vi "FileBLFOpen.vi"(6 "提示语":refnum<vi>, 7 "Language":u32, 8 "进度条":refnum<vi>, 9 "进度数值":refnum<vi>, 10 "报文行数统计":refnum<vi>, 11 "file path (dialog if empty)":path caption="文件路径 （空时为对话框）") -> (0 "路径输出":path, 1 "重构的Data数组":u32[][](array[numeric]), 2 "统计数量":string[](array[string]), 3 "报文ID":string[](array[string]), 4 "基时间簇":T1 {"基时间秒" format="%#.6f"}, 5 "CAN报文统计":string[][](array[string]))   [LabVIEW 2015]
uses:
  BLF/Read Write BLF.lvclass/Read Write BLF.ctl
  GetBinlogdllpath.vi
  BasicAppPath.vi
  <vilib>/Utility/libraryn.llb/Check if File or Folder Exists.vi
  <vilib>/Utility/error.llb/Error Cluster From Error Code.vi
  BLF/Read Write BLF.lvclass
panel:
  out "Object Count":u32
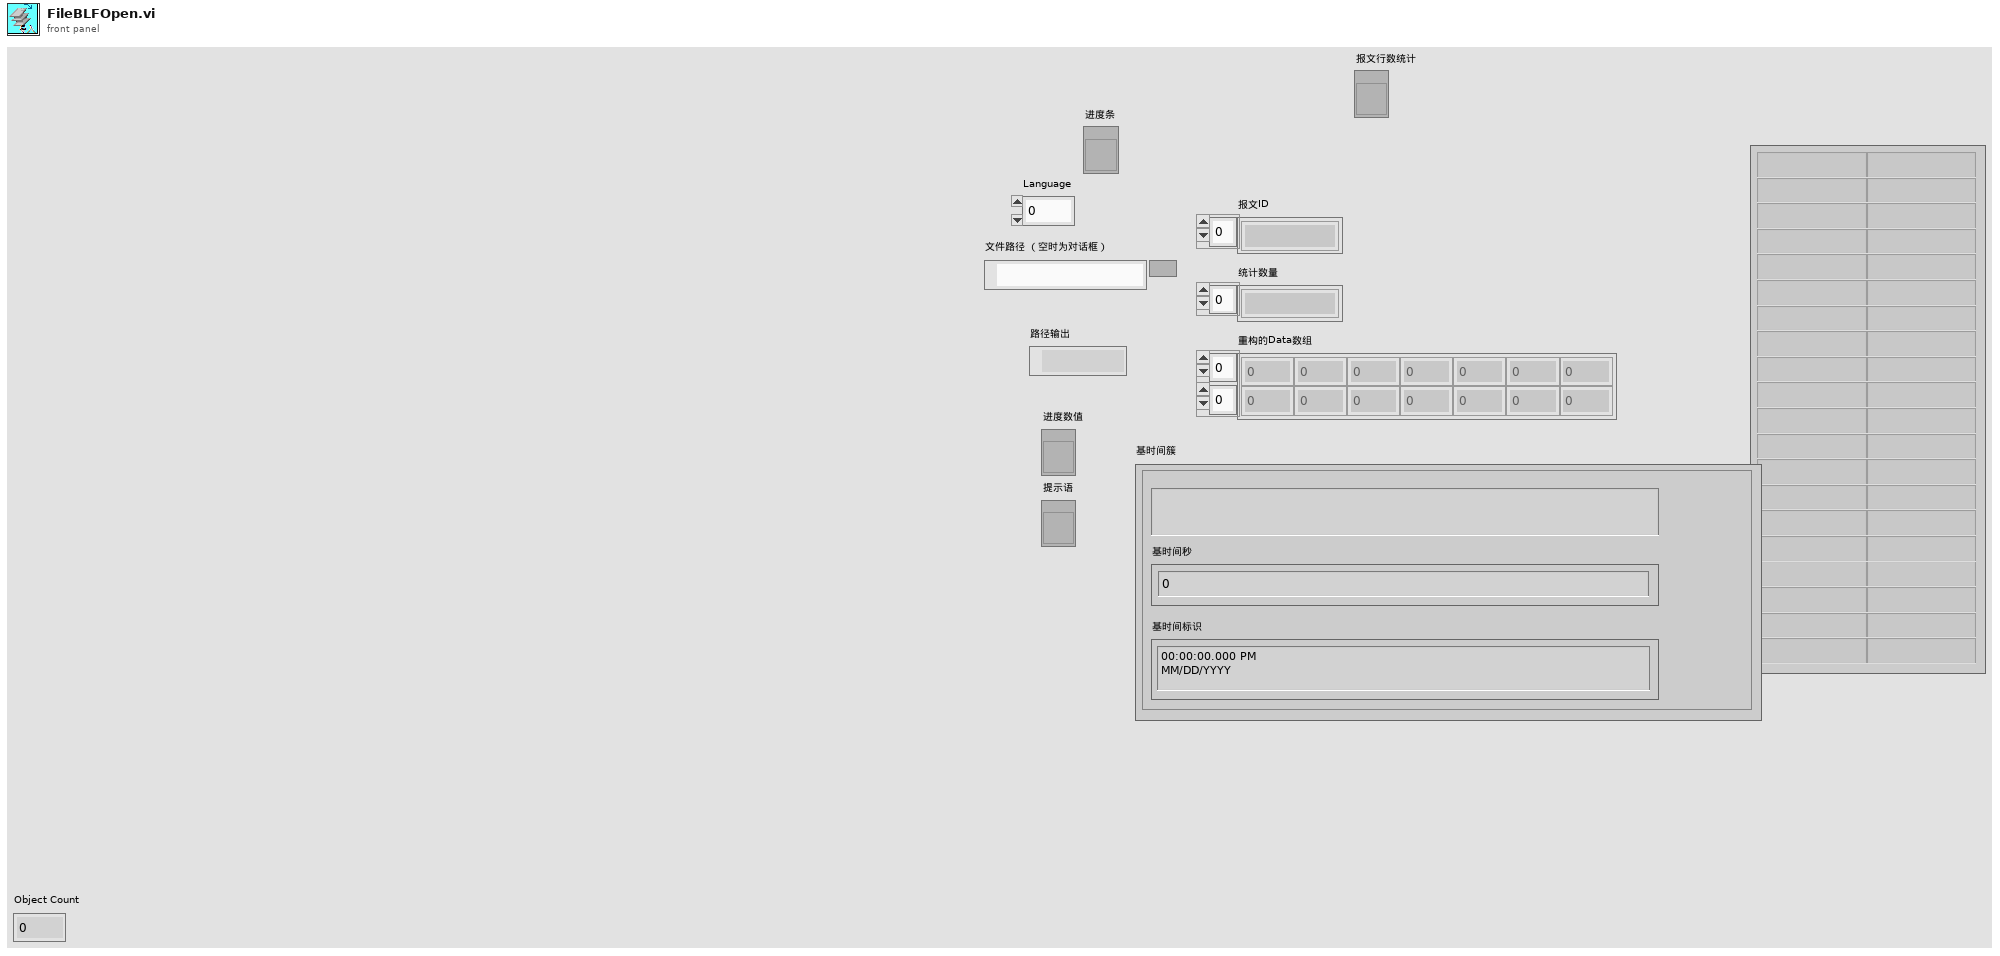
[diagram p1: front panel]
types:
  T1 = cluster{"基时间字符串":string, "基时间秒":dbl, "基时间标识":timestamp}
  T2 = typedef "Read Write BLF.lvclass/Cluster - CAN Frame.ctl" = cluster{"timestamp":timestamp, "payload":u8[], "identifier":u32, "extended?":bool, "echo?":bool, "type":T3}
  T3 = typedef "Read Write BLF.lvclass/Enum - CAN Data Type.ctl" = u8
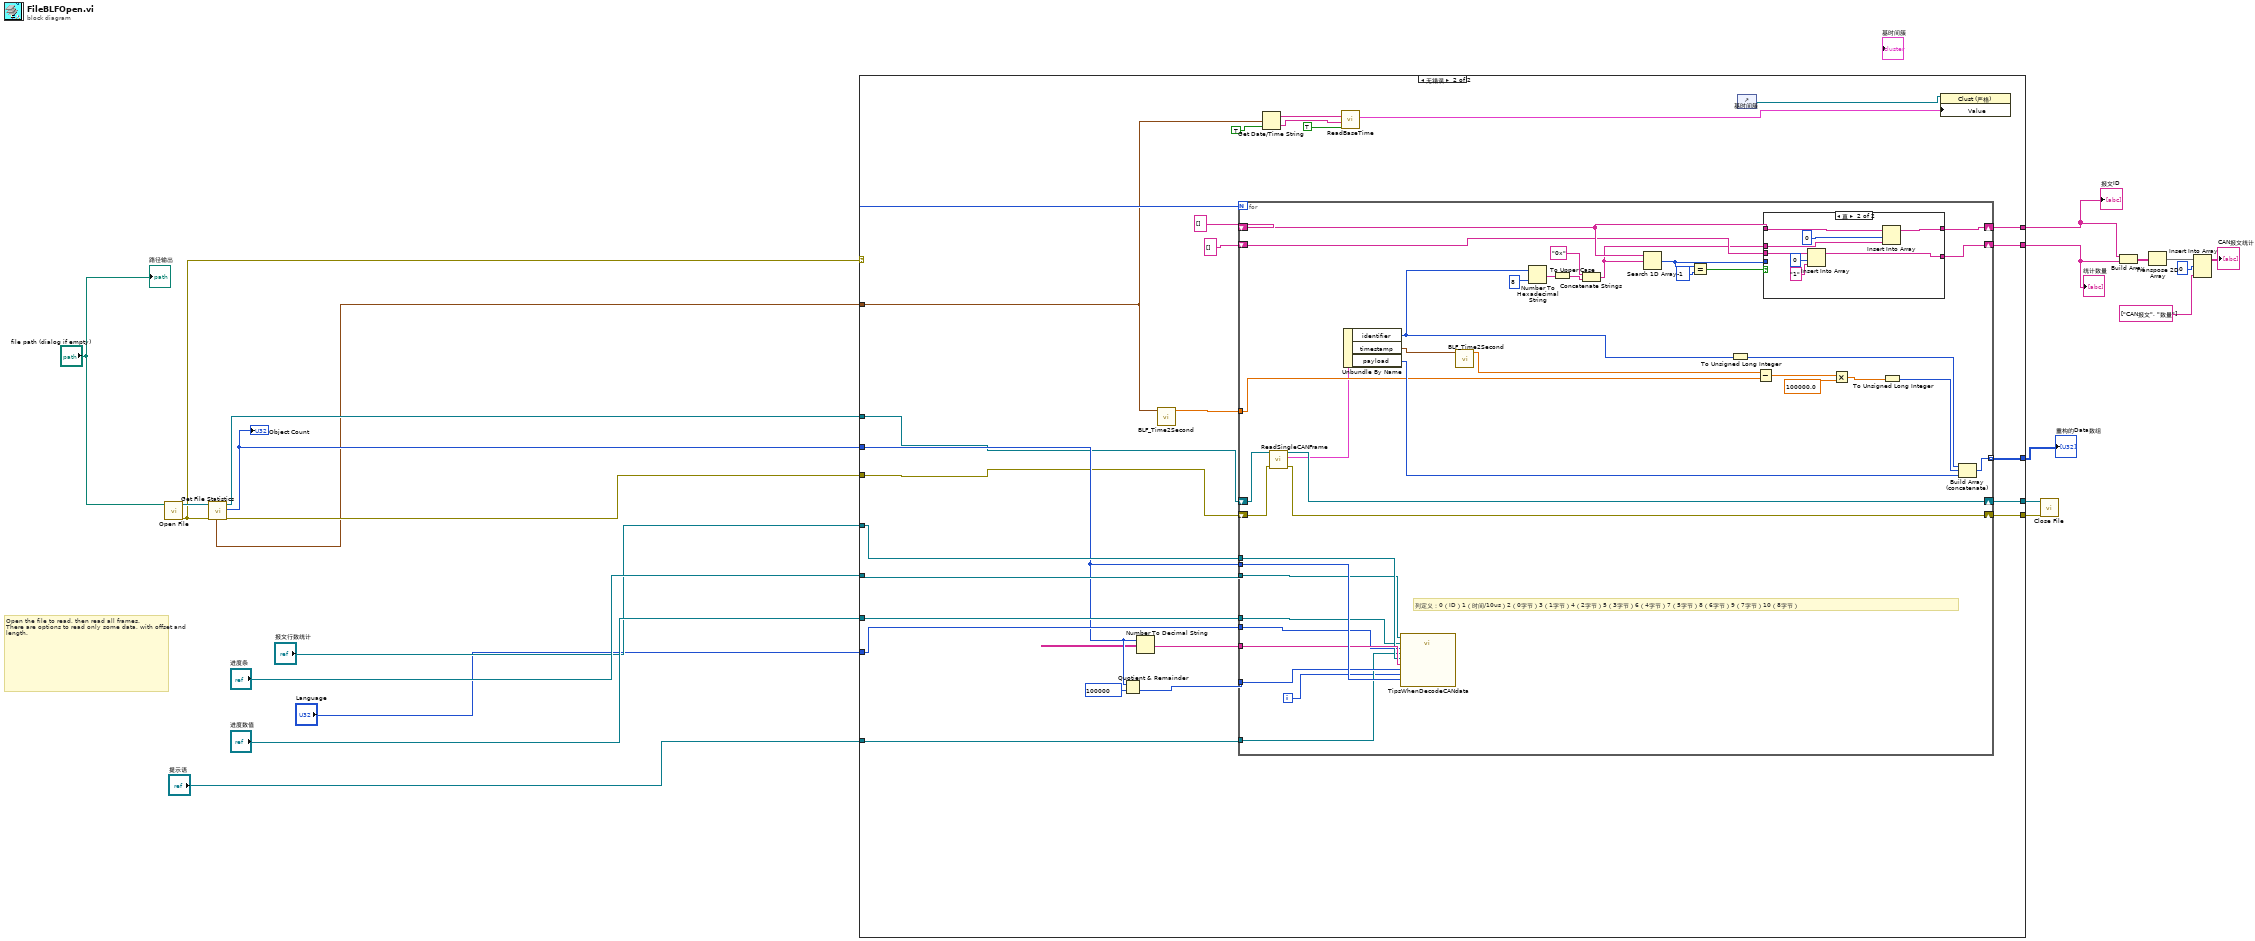
[diagram p0: block diagram]
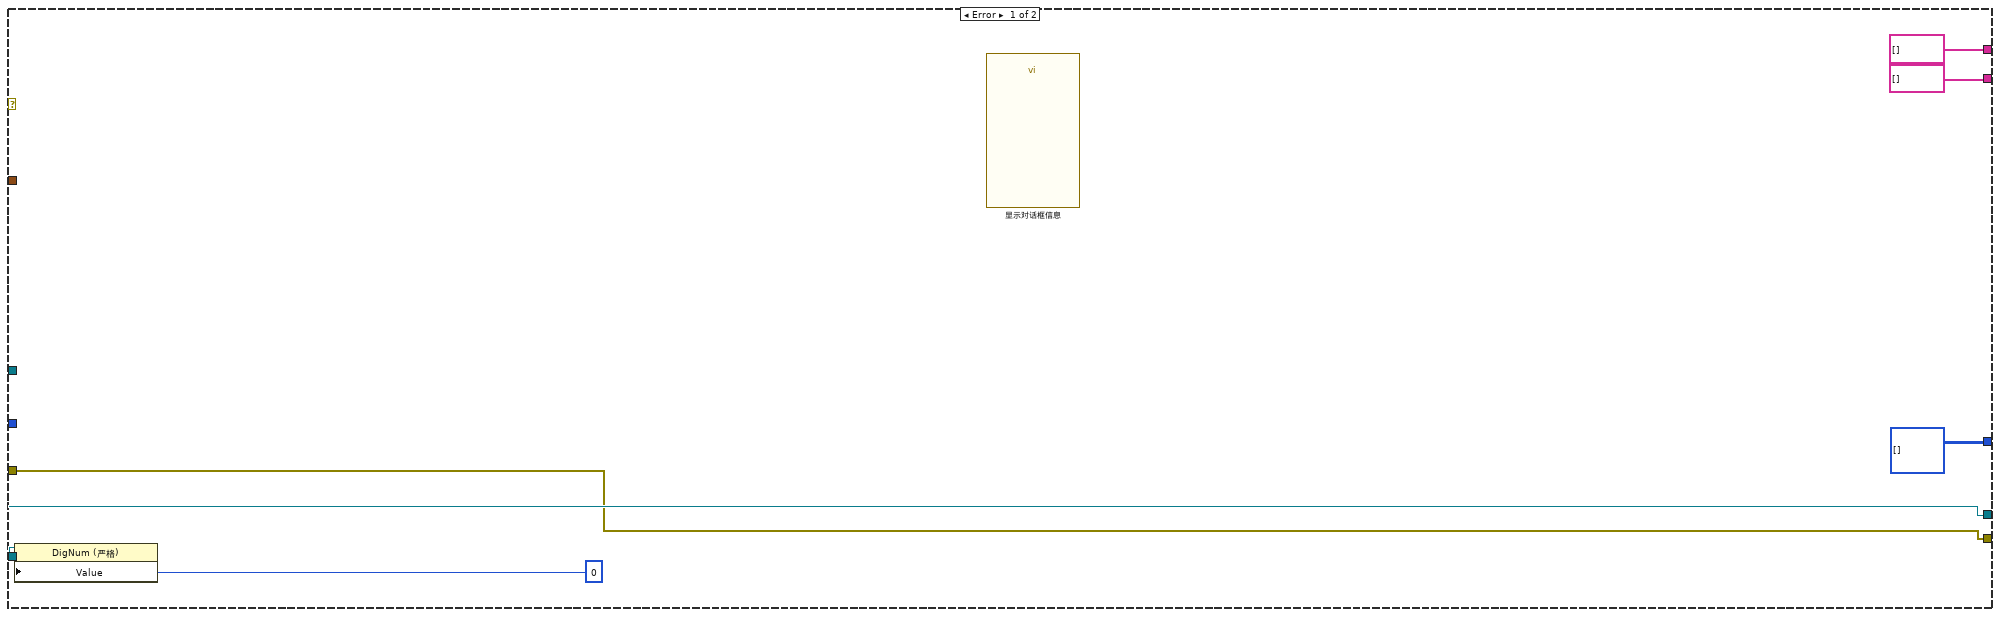
[diagram p2: hidden frame]
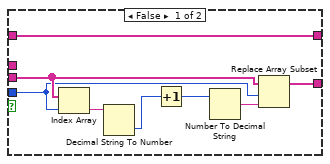
[diagram p3: hidden frame]
diagram:
  # "Open the file to read, then read all frames.\nThere are options to read only some data, with offset and length."
  n1 = call "Open File.vi"("Log Path"="file path (dialog if empty)") -> ("error out"=w8:errorcluster, "BLF File"=w10:refnum<class "Read Write BLF.lvclass">)  [unwired: 9 in]
  n2 = call "Get File Statistics.vi"("error in (no error)"=w8, "Read Write BLF in"=w10) -> ("error out"=w4:errorcluster, "Object Count"=w6:u32, "Read Write BLF out"=w5:refnum<class "Read Write BLF.lvclass">, "Start Time"=w3:timestamp)  [unwired: 3 in, 3 out]
  "Object Count" <- w6
  n3 = case shown="无错误" w8 {
    tunnel: [u32[][] [] w55] -> w22
    tunnel: [string[] [] w52] -> w17
    tunnel: [string[] [] w51] -> w16
    tunnel: "进度条" -> [_ w50]
    tunnel: "进度数值" -> [_ w49]
    tunnel: "提示语" -> [_ w37]
    tunnel: "报文行数统计" -> [w26 w45]
    tunnel: "Language" -> [_ w44]
    tunnel: w6 -> [_ w43]
    tunnel: w5 -> [w24 w32]
    tunnel: w4 -> [w23 w30]
    tunnel: w3 -> [_ w34]
    tunnel: [w24 w33] -> w2
    tunnel: [w23 w31] -> w1
    frame Error {
      n4 = property class="DigNum (严格)"(reference=w26, "Value"=0 ("值")) -> ()  [unwired: 1 in, 2 out]
      n5 = call "显示对话框信息"() -> ()  [unwired: 10 in, 2 out]
    }
    frame No Error {
      n6 = Quotient & Remainder(x=w43, y=100000) -> (floor(x/y)=w47:u32)  [unwired: 1 out]
      n7 = Number To Decimal String(number=w43) -> (decimal integer string=w36:string)  [unwired: 1 in]
      n8 = call "BLF_Time2Second.vi"("Time"=w34) -> ("Second"=w35:dbl)  [unwired: 10 in]
      n9 = for {
        N: w43 -> [_]
        tunnel: [w92] -> w55 mode=indexing
        shift-right: [w87] -> w52
        shift-left: string[] [] -> [w88]
        shift-right: [w83] -> w51
        shift-left: string[] [] -> [w84]
        tunnel: w43 -> [w75]
        tunnel: w50 -> [w68]
        tunnel: w49 -> [w69]
        tunnel: w47 -> [w74]
        tunnel: w37 -> [w71]
        tunnel: w36 -> [w73]
        tunnel: w45 -> [w72]
        tunnel: w44 -> [w70]
        tunnel: w35 -> [w64]
        shift-right: [w60] -> w33
        shift-left: w32 -> [w58]
        shift-right: [w59] -> w31
        shift-left: w30 -> [w57]
        i -> [w63]
        # "列定义：0（ID）1（时间/10us）2（0字节）3（1字节）4（2字节）5（3字节）6（4字节）7（5字节）8（6字节）9（7字节）10（8字节）"
        n10 = call "ReadSingleCANFrame.vi"("error in (no error)"=w57, "BLF File In"=w58) -> ("error out"=w59:errorcluster, "CAN Frame"=w56:T2, "BLF File Out"=w60:refnum<class "Read Write BLF.lvclass">)  [unwired: 6 in, 1 out]
        n11 = Unbundle By Name(w56) -> ("identifier"=w67:u32, "timestamp"=w62:timestamp, "payload"=w66:u8[])
        n12 = call "TipsWhenDecodeCANdata.vi"("ProgressBar"=w68, "AllRowsNum"=w75, "i"=w63, "ProgressNum"=w69, "Language"=w70, "Tips"=w71, "MessageLinCnt"=w72, "txtAllRowsNum"=w73, "RowsLevel"=w74) -> ()  [unwired: 7 in]
        n13 = call "BLF_Time2Second.vi"("Time"=w62) -> ("Second"=w61:dbl)  [unwired: 10 in]
        n14 = Number To Hexadecimal String(1:i16 8 ("宽度(-)"), 2:w67) -> (0:w77:string)
        n15 = To Upper Case(1:w77) -> (0:w76:string)
        n16 = Concatenate Strings("0x" ("字符串"), w76) -> (w79:string)
        n17 = Search 1D Array(1D array=w88, element=w79) -> (index of element=w82:i32)  [unwired: 1 in]
        n18 = Equal?(x=w82, y=-1) -> (x = y?=w85:bool)
        n19 = To Unsigned Long Integer(number=w67) -> (unsigned 32bit integer=w78:u32)
        n20 = Subtract(x=w61, y=w64) -> (x-y=w65:dbl)
        n21 = case shown="真" w85 {
          tunnel: w88 -> [w100 w108]
          tunnel: [w100 w107] -> w87
          tunnel: w79 -> [_ w106]
          tunnel: w84 -> [w99 w103]
          tunnel: [w98 w104] -> w83
          tunnel: w82 -> [w93 _]
          frame False {
            n22 = Index Array(array=w99, index=w93) -> (element=w97:string)
            n23 = Decimal String To Number(string=w97) -> (number=w96:i32)  [unwired: 2 in, 1 out]
            n24 = Increment(x=w96) -> (x+1=w94:i32)
            n25 = Number To Decimal String(number=w94) -> (decimal integer string=w95:string)  [unwired: 1 in]
            n26 = Replace Array Subset(array=w99, new element=w95, index=w93) -> (w98:string[])
          }
          frame True {
            n27 = Insert Into Array(array=w103, index=0 ("索引"), new element="1" ("新元素/子数组")) -> (w104:string[])
            n28 = Insert Into Array(array=w108, index=0 ("索引"), new element=w106) -> (w107:string[])
          }
        }
        n29 = Multiply(x=w65, y=100000.0) -> (x*y=w90:dbl)
        n30 = To Unsigned Long Integer(number=w90) -> (unsigned 32bit integer=w89:u32)
        n31 = Build Array (concatenate)(w78, w89, w66) -> (w92:u32[])
      }
      n32 = Get Date/Time String(seconds (now)=w34, want seconds? (F)=TRUE ("需要秒？(F)")) -> (date string=w41:string, time string=w40:string)  [unwired: 1 in]
      n33 = call "ReadBaseTime.vi"("文件时间？(F)"=TRUE, "时间字符"=w40, "日期字符"=w41) -> ("基时间簇"=w38:T1)  [unwired: 6 in]
      n34 = control-ref of="基时间簇"() -> (w46:refnum<vi>)
      n35 = property class="Clust (严格)"(reference=w46, "Value"=w38) -> ()  [unwired: 1 in, 2 out]
    }
  }
  "重构的Data数组" <- w22
  "报文ID" <- w17
  "统计数量" <- w16
  n36 = call "Close File.vi"("error in (no error)"=w1, "BLF File"=w2) -> ()  [unwired: 8 in, 2 out]
  n37 = Build Array(w17, w16) -> (w21:string[][])
  n38 = Transpose 2D Array(2D array=w21) -> (transposed array=w20:string[][])
  n39 = Insert Into Array(array=w20, index (row)=0 ("索引 (行)"), new element=string[] ["CAN报文", "数量"]) -> (→"CAN报文统计":string[][])  [unwired: 1 in]
  "路径输出" <- "file path (dialog if empty)"
